vi "IPS Read Switch Heater Current.vi"(4 "Error In":errorcluster, 7 "VISA resource name":refnum<visa-resource-name>="GPIB1::25::INSTR") -> (0 "Error Out":errorcluster, 1 "heater current (mA)":dbl, 2 "Response":string, 3 "VISA resource name":refnum<visa-resource-name>)   [LabVIEW 2016, in "IPS-120.lvlib"]
uses:
  IPS-120.lvlib
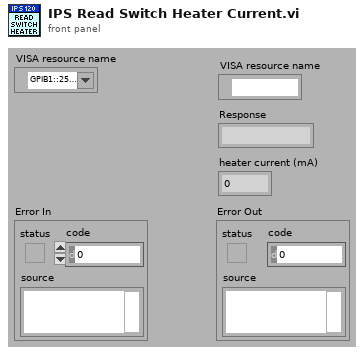
[diagram p1: front panel]
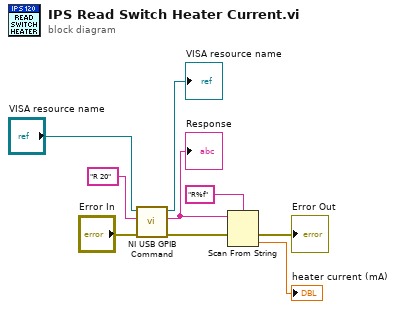
[diagram p0: block diagram]
diagram:
  n1 = call "NI USB GPIB Command.vi"("Error In"="Error In", "write buffer"="R 20" ("String to Send"), "VISA resource name"="VISA resource name") -> ("Error Out"=w3:errorcluster, "read buffer"=w4:string, "VISA resource name out"=→"VISA resource name":refnum<visa-resource-name>)  [unwired: 6 in]
  "Response" <- w4
  n2 = Scan From String(format string="R%f", input string=w4, error in=w3) -> (error out=→"Error Out":errorcluster, output 1=→"heater current (mA)":dbl)  [unwired: 1 in, 3 out]
